vi "rsscope Initiate Acquisition.vi"(8 "error in (no error)":errorcluster, 10 "Action (Single)":i32(ring) items=["Single", "Continuous", "Force", "Single Without Wait"], 11 "VISA resource name":refnum<visa-resource-name>) -> (0 "error out":errorcluster, 3 "VISA resource name out":refnum<visa-resource-name>)   [LabVIEW 2014]
doc: "This VI initiates a waveform acquisition. After you call this VI, the oscilloscope leaves the Idle state and waits for a trigger. The oscilloscope acquires a waveform for each channel you have enabled with the rsscope Configure Channel.vi.\n\nAttributes:\nRSSCOPE_ATTR_RUN_SINGLE\nRSSCOPE_ATTR_RUN_CONTINUOUS\nRSSCOPE_ATTR_FORCE\nRSSCOPE_ATTR_RUN_SINGLE_WITHOUT_WAIT\n\nRemote-control commands:\nSINGle\nRUN\nTRIGger<m>:FORCe"
uses:
  Instance           1 36Saved   rsscope Initiate Acquisition .vi
  Instance           2 36Saved   rsscope Initiate Acquisition .vi
  Instance           3 36Saved   rsscope Initiate Acquisition .vi
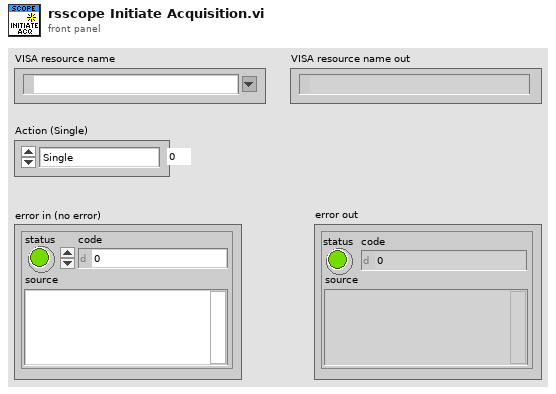
[diagram p1: front panel]
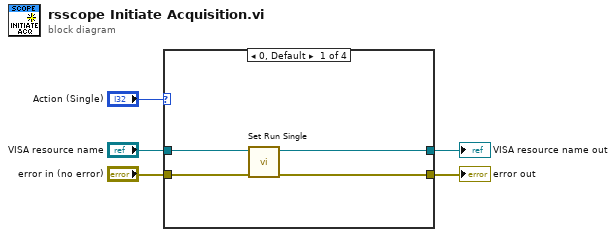
[diagram p0: block diagram]
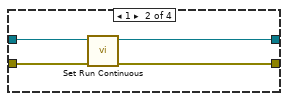
[diagram p2: hidden frame]
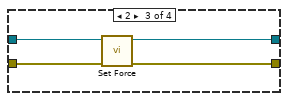
[diagram p3: hidden frame]
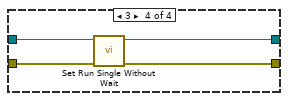
[diagram p4: hidden frame]
diagram:
  n1 = case shown="0, Default" "Action (Single)" {
    tunnel: "error in (no error)" -> [w8 w10 w17 w20]
    tunnel: "VISA resource name" -> [w9 w11 w16 w21]
    tunnel: [w7 w12 w15 w19] -> w3
    tunnel: [w6 w13 w14 w18] -> w2
    frame 0, Default {
      n2 = call "Set Run Single"("error in (no error)"=w8, "instrument handle"=w9) -> ("error out"=w7:errorcluster, "instrument handle out"=w6:refnum<visa-resource-name>)  [unwired: 8 in]
    }
    frame 1 {
      n3 = call "Set Run Continuous"("error in (no error)"=w10, "instrument handle"=w11) -> ("error out"=w12:errorcluster, "instrument handle out"=w13:refnum<visa-resource-name>)  [unwired: 8 in]
    }
    frame 2 {
      n4 = call "Set Force"("error in (no error)"=w17, "instrument handle"=w16) -> ("error out"=w15:errorcluster, "instrument handle out"=w14:refnum<visa-resource-name>)  [unwired: 8 in]
    }
    frame 3 {
      n5 = call "Set Run Single Without Wait"("error in (no error)"=w20, "instrument handle"=w21) -> ("error out"=w19:errorcluster, "instrument handle out"=w18:refnum<visa-resource-name>)  [unwired: 8 in]
    }
  }
  "error out" <- w3
  "VISA resource name out" <- w2
